vi "brc_daq_get_available_ch_names.vi"() -> (14 "available_chs":string[](array[string]))   [LabVIEW 2015, in "BRC-DAQ x64.lvlib"]
uses:
  BRC-DAQ x64.lvlib
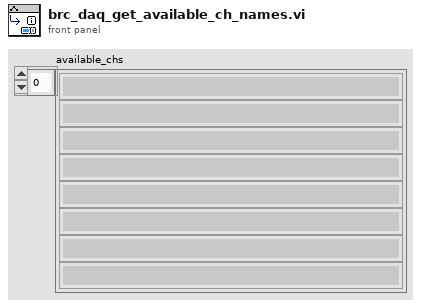
[diagram p1: front panel]
types:
  T1 = typedef "BRC-DAQ x64.lvlib/brc_daq_pModuleInfo.ctl" = cluster{"deviceId":string, "productName":string, "channelCount":i32}
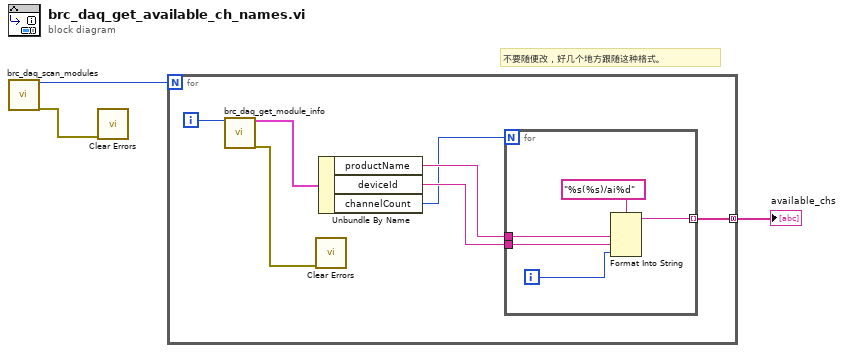
[diagram p0: block diagram]
diagram:
  # "不要随便改，好几个地方跟随这种格式。"
  n1 = call "brc_daq_scan_modules.vi"() -> ("module_number"=w3:i32, "error out"=w1:errorcluster)  [unwired: 18 in]
  n2 = call <vilib>:"Clear Errors.vi"("error in (no error)"=w1) -> ()  [unwired: 5 in, 2 out]
  n3 = for {
    N: w3 -> [_]
    tunnel: [w5] -> w2 mode=concatenating
    i -> [w10]
    n4 = call "brc_daq_get_module_info.vi"("index"=w10) -> ("pModuleInfo_cluster"=w9:T1, "error out"=w4:errorcluster)  [unwired: 17 in]
    n5 = call <vilib>:"Clear Errors.vi"("error in (no error)"=w4) -> ()  [unwired: 5 in, 2 out]
    n6 = Unbundle By Name(w9) -> ("productName"=w8:string, "deviceId"=w7:string, "channelCount"=w6:i32)
    n7 = for {
      N: w6 -> [_]
      tunnel: w8 -> [w12]
      tunnel: w7 -> [w11]
      tunnel: [w13] -> w5 mode=indexing
      i -> [w14]
      n8 = Format Into String(format string="%s(%s)/ai%d", w12, w11, w14) -> (resulting string=w13:string)  [unwired: 2 in, 1 out]
    }
  }
  "available_chs" <- w2
